vi "createFITSfile.vi"(8 "error in (no error)":errorcluster, 10 "Path":path=path "!/home/harini/TCS/SEDSpectrum", 11 "Model in":refnum<class "Model.lvclass">) -> (0 "error out":errorcluster, 3 "Model out":refnum<class "Model.lvclass">)   [LabVIEW 2016, in "Model.lvclass"]
uses:
  Model.lvclass
  Model.lvclass/Model.ctl
  CFitsIO/CFitsIO.lvclass
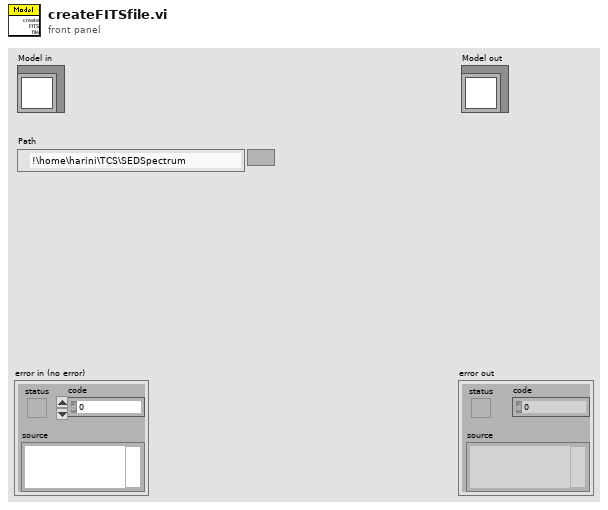
[diagram p1: front panel]
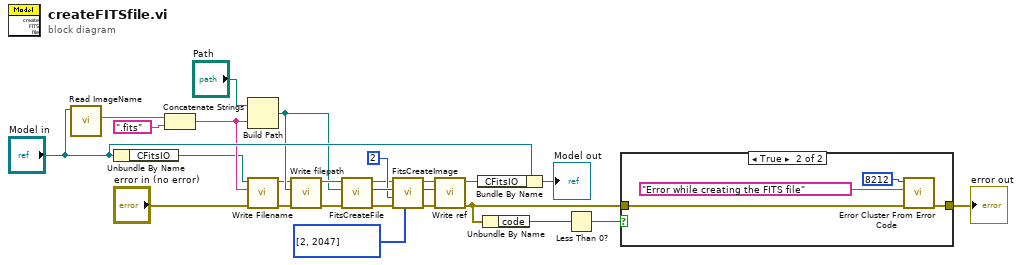
[diagram p0: block diagram]
diagram:
  n1 = call-dynamic "Read ImageName.vi"("Model in"="Model in") -> ("ImageName"=w22:string)  [unwired: 8 in, 2 out]
  n2 = Unbundle By Name("Model in") -> ("CFitsIO"=w4:refnum<class "CFitsIO.lvclass">)
  n3 = Concatenate Strings(w22, ".fits" ("string")) -> (w5:string)
  n4 = Build Path(base path="Path", name or relative path=w5) -> (appended path=w10:path)
  n5 = call-dynamic "Write Filename.vi"("error in (no error)"="error in (no error)", "Filename"=w5, "CFitsIO in"=w4) -> ("error out"=w1:errorcluster, "CFitsIO out"=w3:refnum<class "CFitsIO.lvclass">)  [unwired: 7 in]
  n6 = call-dynamic "Write filepath.vi"("error in (no error)"=w1, "Filepath"=w10, "CFitsIO in"=w3) -> ("error out"=w12:errorcluster, "CFitsIO out"=w11:refnum<class "CFitsIO.lvclass">)  [unwired: 7 in]
  n7 = call-dynamic "FitsCreateFile.vi"("error in (no error)"=w12, "Path"=w10, "CFitsIO in"=w11) -> ("error out"=w17:errorcluster, "fd"=w20:u64, "CFitsIO out"=w15:refnum<class "CFitsIO.lvclass">)  [unwired: 5 in, 1 out]
  n8 = call-dynamic "FitsCreateImage.vi"("naxes"=i64[] [2, 2047], "error in (no error)"=w17, "naxis"=2, "ref in"=w20, "CFitsIO in"=w15) -> ("error out"=w16:errorcluster, "ref out"=w19:u64, "CFitsIO out"=w14:refnum<class "CFitsIO.lvclass">)  [unwired: 4 in]
  n9 = call-dynamic "Write ref .vi"("error in (no error)"=w16, "ref"=w19, "CFitsIO in"=w14) -> ("error out"=w7:errorcluster, "CFitsIO out"=w26:refnum<class "CFitsIO.lvclass">)  [unwired: 7 in]
  n10 = Bundle By Name(cluster="Model in", "CFitsIO"=w26) -> (→"Model out":refnum<class "Model.lvclass">)
  n11 = Unbundle By Name(w7) -> ("code"=w9:i32)
  n12 = Less Than 0?(x=w9) -> (x < 0?=w8:bool)
  n13 = case shown="True" w8 {
    tunnel: [w27 w29] -> w6
    tunnel: w7 -> [w27 w28]
    frame False {
    }
    frame True {
      n14 = call <vilib>:"Error Cluster From Error Code.vi"("error in (no error)"=w28, "error message (\"\")"="Error while creating the FITS file" ("error message (\"\")"), "error code (0)"=8212) -> ("error out"=w29:errorcluster)  [unwired: 6 in]
    }
  }
  "error out" <- w6
